vi "Testcode.vi"() -> ()   [LabVIEW 2021]
uses:
  MallardDuck/MallardDuck.lvclass
  Duck/Duck.lvclass
panel:
  out "error out":errorcluster
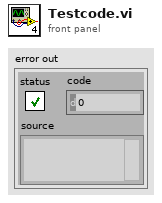
[diagram p1: front panel]
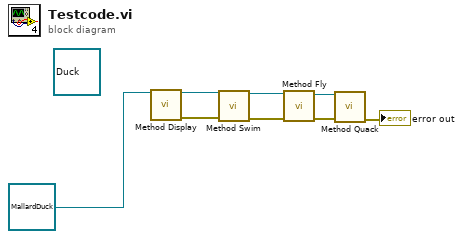
[diagram p0: block diagram]
diagram:
  (unwired) refnum<class "Duck.lvclass"> refnum ("Duck.lvclass")
  n1 = call-dynamic "Method Display.vi"("Duck in"=refnum<class "MallardDuck.lvclass"> refnum ("MallardDuck.lvclass")) -> ("Duck out"=w6:refnum<class "MallardDuck.lvclass">, "error out"=w8:errorcluster)  [unwired: 13 in]
  n2 = call-dynamic "Method Swim.vi"("Duck in"=w6, "error in (no error)"=w8) -> ("Duck out"=w5:refnum<class "MallardDuck.lvclass">, "error out"=w7:errorcluster)  [unwired: 12 in]
  n3 = call-dynamic "Method Fly.vi"("error in (no error)"=w7, "Duck in"=w5) -> ("error out"=w3:errorcluster, "Duck out"=w4:refnum<class "MallardDuck.lvclass">)  [unwired: 8 in]
  n4 = call-dynamic "Method Quack.vi"("MallardDuck in"=w4, "error in (no error)"=w3) -> ("error out"=→"error out":errorcluster)  [unwired: 12 in, 1 out]
